vi "Module Name--constant.vi"() -> (3 "Module Name":string)   [LabVIEW 2020, in "Wordle Engine.lvlib"]
doc: "Return the name of the module that owns this VI. \n_____\nBased on DQMH Project Template 6.1.0.93."
uses:
  Wordle Engine.lvlib
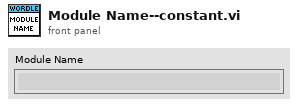
[diagram p1: front panel]
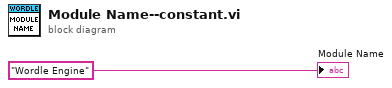
[diagram p0: block diagram]
diagram:
  "Module Name" <- "Wordle Engine"
